vi "get flattened children.vi"(8 "error in":errorcluster, 10 "ID":string, 11 "flat hierarchy":T2) -> (0 "error out":errorcluster, 1 "children":T1[](array[typedef]))   [LabVIEW 2013, in "NISE_CEF_TreeSerializer.lvlib"]
uses:
  NISE_CEF_TreeSerializer.lvlib
  flat hierarchy.ctl
  full hierarchy.ctl
  hierarchy element.ctl
  instance data.ctl
  NISE_CEF_TreeControl.lvlib
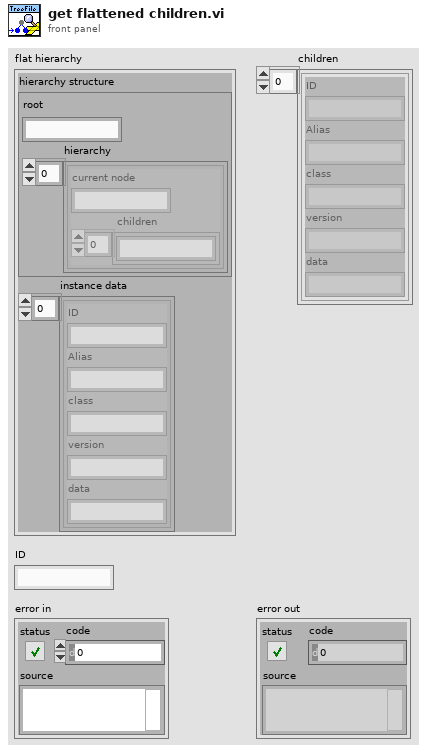
[diagram p1: front panel]
types:
  T1 = typedef "NISE_CEF_TreeSerializer.lvlib/instance data.ctl" = cluster{"ID":string, "Alias":string, "class":string, "version":string, "data":string}
  T2 = typedef "NISE_CEF_TreeSerializer.lvlib/flat hierarchy.ctl" = cluster{"hierarchy structure":T3, "instance data":T1[]}
  T3 = typedef "NISE_CEF_TreeSerializer.lvlib/full hierarchy.ctl" = cluster{"root":string, "hierarchy":T4[]}
  T4 = typedef "NISE_CEF_TreeSerializer.lvlib/hierarchy element.ctl" = cluster{"current node":string, "children":string[]}
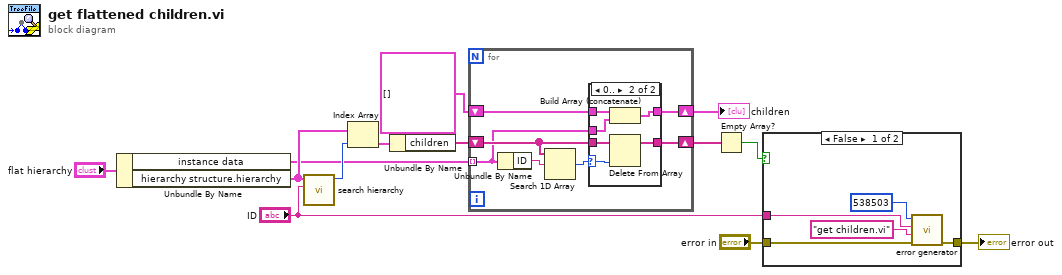
[diagram p0: block diagram]
diagram:
  n1 = Unbundle By Name("flat hierarchy") -> ("instance data"=w9:T1[], "hierarchy structure.hierarchy"=w12:T4[])
  n2 = call "search hierarchy.vi"("ID"="ID", "hierarchy"=w12) -> ("index"=w11:i32)  [unwired: 9 in]
  n3 = Index Array(array=w12, index=w11) -> (element=w10:T4)
  n4 = Unbundle By Name(w10) -> ("children"=w8:string[])
  n5 = for {
    tunnel: w9 -> [w14] mode=indexing
    shift-right: [w16] -> w4
    shift-left: w8 -> [w17]
    shift-right: [w19] -> w6
    shift-left: T1[] [] -> [w18]
    n6 = Unbundle By Name(w14) -> ("ID"=w15:string)
    n7 = Search 1D Array(1D array=w17, element=w15) -> (index of element=w20:i32)  [unwired: 1 in]
    n8 = case shown="0.." w20 {
      selector: w20 -> [_ w24]
      tunnel: w14 -> [_ w28]
      tunnel: [w22 w27] -> w19
      tunnel: w18 -> [w22 w26]
      tunnel: w17 -> [w21 w25]
      tunnel: [w21 w23] -> w16
      frame ..-1 {
      }
      frame 0.. {
        n9 = Build Array (concatenate)(w26, w28) -> (w27:T1[])
        n10 = Delete From Array(array=w25, index=w24) -> (array with subset deleted=w23:string[])  [unwired: 1 in, 1 out]
      }
    }
  }
  "children" <- w6
  n11 = Empty Array?(array=w4) -> (empty?=w3:bool)
  n12 = case shown="False" w3 {
    tunnel: "ID" -> [w31 _]
    tunnel: "error in" -> [w30 w34]
    tunnel: [w29 w34] -> w1
    frame False {
      n13 = call "error generator.vi"("error in"=w30, "source"="get children.vi", "append error message"=w31, "error code (0)"=538503) -> ("error out"=w29:errorcluster)  [unwired: 5 in]
    }
    frame True {
    }
  }
  "error out" <- w1
